vi "ClearNetworkStreamNotConnectedError.vi"(11 "ErrorIn":errorcluster) -> (3 "ErrorOut":errorcluster)   [LabVIEW 2018]
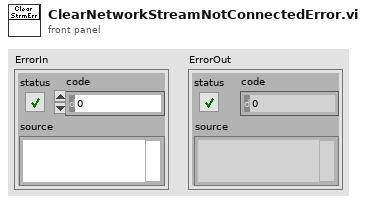
[diagram p1: front panel]
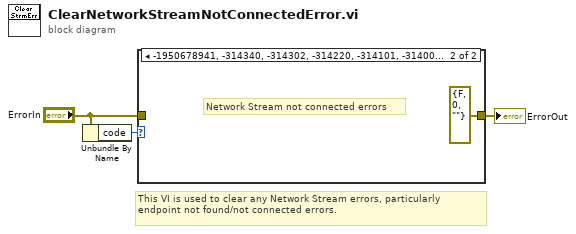
[diagram p0: block diagram]
diagram:
  # "This VI is used to clear any Network Stream errors, particularly endpoint not found/not connected errors."
  n1 = Unbundle By Name("ErrorIn") -> ("code"=w3:i32)
  n2 = case shown="-1950678941, -314340, -314302, -314220, -314101, -314004" w3 {
    tunnel: [w4 errorcluster {"status"=FALSE, "code"=0, "source"=""} ("ErrorIn")] -> w1
    tunnel: "ErrorIn" -> [w4 _]
    frame Default {
      # "All other errors"
    }
    frame -1950678941, -314340, -314302, -314220, -314101, -314004 {
      # "Network Stream not connected errors"
    }
  }
  "ErrorOut" <- w1
